vi "graph temp and power.vi"(0 "Temperature Graph":refnum<vi>, 7 "temp":T3 {"utility"."therm volt" format="%_6g"; "utility"."heat volt in" format="%_6g"; "utility"."heat volt out" format="%_6g"; "utility"."power out" format="%_6g"; "utility"."H Vmax" format="%_6g"; "T exec"."man power" format="%_6g"; "T exec"."exec setpoint" format="%_6g"; "T params"."Settle Time" step=1.0; "T params"."Settle Bandwidth" step=0.01; "T params"."Derivative Tme" step=0.01; "T params"."Integral Time" step=1.0; "T params"."Control Bandwidth" step=0.1; "T params"."Setpoint" step=0.1; "T status"."Setpoint" format="%_6g"; "T status"."Power" format="%_6g"; "T status"."Temp" format="%_6g"}, 11 "show power":bool) -> (2 "meas index":i32, 3 "latest time (s)":dbl, 4 "man":bool, 8 "T and P graph":cluster{"t hist":dbl[], "T hist":dbl[]}[](array[cluster]), 15 "T status":T1 {"Setpoint" format="%_6g"; "Power" format="%_6g"; "Temp" format="%_6g"})   [LabVIEW 2019]
doc: "This is a Bug C(T) subVI.\n\nThis subVI manages the data extraction for the time, temperature, and power for the full history graph in the bug experiment. It scales the normalized power to the given temperature scale of the graph dynamically.\n\nPaul K Dixon\nP3600\nCSUSB Physics"
uses:
  typedefs/temp cont cluster.ctl
  typedefs/temp exec cluster.ctl
  typedefs/temp mode enum.ctl
  typedefs/temp indicator.ctl
  typedefs/temp control status.ctl
  typedefs/PID control parameters.ctl
  typedefs/temp cont utility.ctl
panel:
  out "P plot":cluster{"t hist":dbl[], dbl[]}
  out "T plot":cluster{"t hist":dbl[], "T hist":dbl[]}
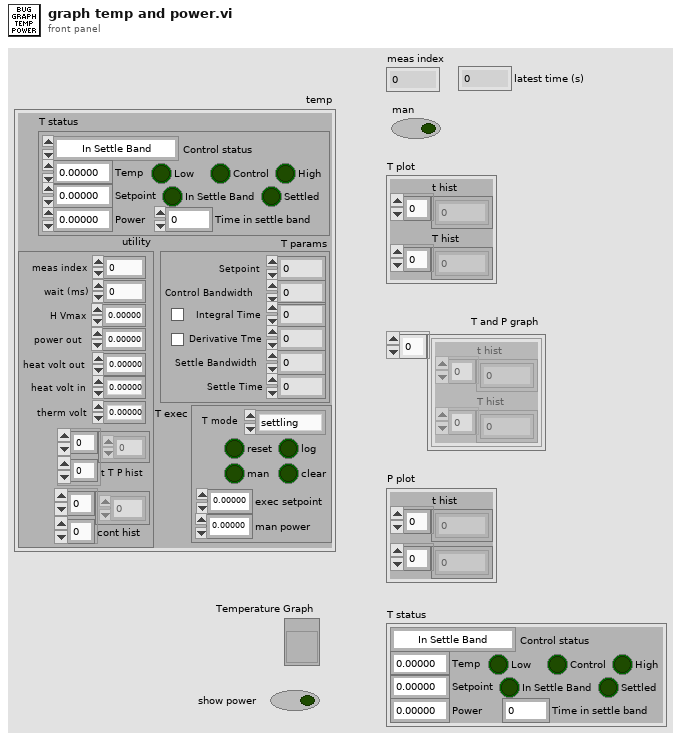
[diagram p1: front panel]
types:
  T1 = typedef "temp indicator.ctl" = cluster{"Control status":T2, "Temp":dbl, "Power":dbl, "Time in settle band":dbl, "Settled":bool, "Low":bool, "High":bool, "Setpoint":dbl, "Control":bool, "In Settle Band":bool}
  T2 = typedef "temp control status.ctl" = enum16{"In Settle Band", "In Control Band", "Below Control Band", "Above Control Band"}
  T3 = typedef "temp cont cluster.ctl" = cluster{"T exec":T4, "T status":T1, "T params":T6, "utility":T7}
  T4 = typedef "temp exec cluster.ctl" = cluster{"T mode":T5, "exec setpoint":dbl, "reset":bool, "man power":dbl, "man":bool, "log":bool, "clear":bool}
  T5 = typedef "temp mode enum.ctl" = enum16{"settling", "measuring", "holding", "Exit"}
  T6 = typedef "PID control parameters.ctl" = cluster{"Setpoint":dbl, "Control Bandwidth":dbl, "Integral Time":dbl, "Int\nON":bool, "Derivative Tme":dbl, "Der\nON":bool, "Settle Bandwidth":dbl, "Settle Time":dbl}
  T7 = typedef "temp cont utility.ctl" = cluster{"meas index":i32, "wait (ms)":i32, "H Vmax":dbl, "power out":dbl, "heat volt out":dbl, "heat volt in":dbl, "therm volt":dbl, "t T P hist":dbl[][], "cont hist":dbl[][]}
  T8 = cluster{"t T P hist":dbl[], "t T P hist":dbl[]}[]
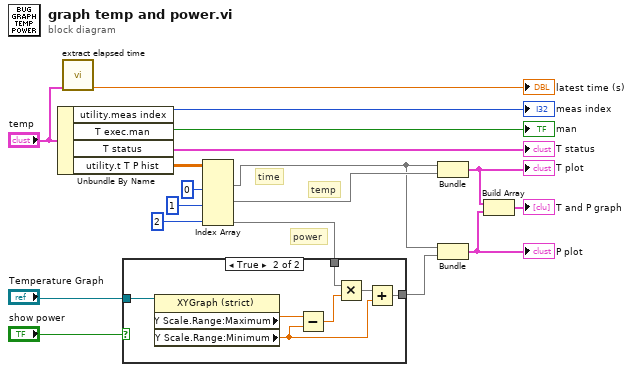
[diagram p0: block diagram]
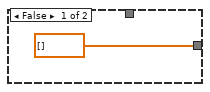
[diagram p2: hidden frame]
diagram:
  # "power"
  # "temp"
  # "time"
  n1 = Unbundle By Name("temp") -> ("utility.meas index"=→"meas index":i32, "T exec.man"=→"man":bool, "T status"=→"T status":T1, "utility.t T P hist"=w14:dbl[][])
  n2 = call "extract elapsed time.vi"("temp"="temp") -> ("latest time (s)"=→"latest time (s)":dbl)  [unwired: 14 in]
  n3 = Index Array(array=w14, index (col) #1=0 ("disabled index (col)"), index (col) #2=1 ("index (col)"), index (col) #3=2 ("index (col)")) -> (element #1=w11:dbl[], element #2=w13:dbl[], element #3=w12:dbl[])  [unwired: 3 in]
  n4 = case shown="True" "show power" {
    tunnel: [dbl[] [] w22] -> w16
    tunnel: "Temperature Graph" -> [_ w21]
    tunnel: w12 -> [_ w20]
    frame False {
    }
    frame True {
      n5 = property class="XYGraph (strict)"(reference=w21) -> ("Y Scale.Range:Maximum"=w26:dbl, "Y Scale.Range:Minimum"=w25:dbl)  [unwired: 1 in, 2 out]
      n6 = Subtract(x=w26, y=w25) -> (x-y=w23:dbl)
      n7 = Multiply(x=w20, y=w23) -> (x*y=w24:dbl[])
      n8 = Add(x=w24, y=w25) -> (x+y=w22:dbl[])
    }
  }
  n9 = Bundle("t T P hist"=w11, "t T P hist"=w13) -> (w9:cluster{"t T P hist":dbl[], "t T P hist":dbl[]})  [unwired: 1 in]
  "T plot" <- w9
  n10 = Bundle("t T P hist"=w11, w16) -> (w8:cluster{"t T P hist":dbl[], dbl[]})  [unwired: 1 in]
  "P plot" <- w8
  n11 = Build Array(w9, w8) -> (→"T and P graph":T8)
